vi "Main VI.vi"(8 "error in (no error)":errorcluster) -> (0 "error out":errorcluster, 3 "Boolean":bool)   [LabVIEW 2023, in "Error Handling.lvlib"]
doc: "Hanldes the possible errors that could arrive.\nIf no initial enter manu mode frame is entered or if the heartbeat stops, send signals to ingress to normal mode"
uses:
  Error Handling.lvlib
  Internal Communication/Internal Communication.lvlib
panel:
  out "State":string
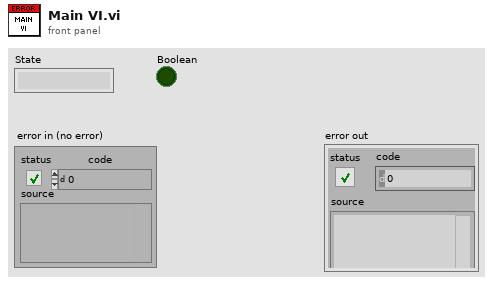
[diagram p1: front panel]
types:
  T1 = typedef "Queue.ctl" = refnum<queue>
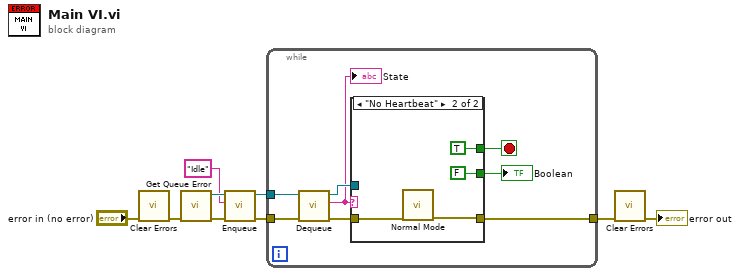
[diagram p0: block diagram]
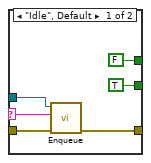
[diagram p2: hidden frame]
diagram:
  n1 = call <vilib>:"Clear Errors.vi"("error in (no error)"="error in (no error)") -> ("error out"=w6:errorcluster)  [unwired: 5 in, 1 out]
  n2 = call "Get Queue Error.vi"("error in (no error)"=w6) -> ("error out"=w5:errorcluster, "Error Queue"=w4:refnum<queue>)  [unwired: 8 in, 1 out]
  n3 = call "Enqueue.vi"("error in (no error)"=w5, "Command"="Idle", "Queue In"=w4) -> ("error out"=w2:errorcluster, "Queue Out"=w1:T1)  [unwired: 7 in]
  n4 = while {
    tunnel: [w17] -> w8
    tunnel: w2 -> [w14]
    tunnel: w1 -> [w13]
    stop <- w16 stop-if-true
    n5 = call "Dequeue.vi"("error in (no error)"=w14, "Queue In"=w13) -> ("error out"=w12:errorcluster, "String"=w10:string, "Queue Out"=w11:T1)  [unwired: 6 in, 1 out]
    "State" <- w10
    n6 = case shown="\"No Heartbeat\"" w10 {
      selector: w10 -> [w18 _]
      tunnel: [FALSE TRUE ("Boolean 2")] -> w16
      tunnel: [w21 w24] -> w17
      tunnel: [TRUE ("Boolean 2") FALSE ("Boolean 2")] -> w15
      tunnel: w12 -> [w20 w25]
      tunnel: w11 -> [w19 _]
      frame "Idle", Default {
        n7 = call "Enqueue.vi"("error in (no error)"=w20, "Command"=w18, "Queue In"=w19) -> ("error out"=w21:errorcluster)  [unwired: 7 in, 1 out]
      }
      frame "No Heartbeat" {
        n8 = call "Normal Mode.vi"("error in (no error)"=w25) -> ("error out"=w24:errorcluster)  [unwired: 10 in]
      }
    }
    "Boolean" <- w15
  }
  n9 = call <vilib>:"Clear Errors.vi"("error in (no error)"=w8) -> ("error out"=→"error out":errorcluster)  [unwired: 5 in, 1 out]
